vi "CD Engine lvlib.vi"(9 "Action":T1) -> (1 "Output":string)   [LabVIEW 2015, in "NIVS_Consolidated_CDW_MetaDataObj.lvclass"]
doc: "Constants, which are necessary for the <B>CD Engine library</B> in the generated custom device project."
uses:
  NIVS_Consolidated_CDW_MetaDataObj.lvclass
  CD Engine lvlib.ctl
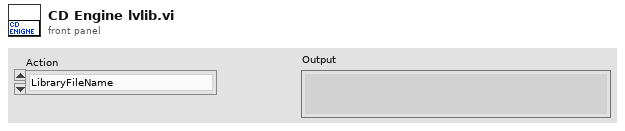
[diagram p1: front panel]
types:
  T1 = typedef "NIVS_Consolidated_CDW_MetaDataObj.lvclass/CD Engine lvlib.ctl" = enum16{"LibraryFileName", "LibraryFolderName", "Engine.FolderName", "Engine.Init.FolderName", "Engine.Run.FolderName", "Engine.Shutdown.FolderName", "Types.FolderName", "Engine.RT Driver VI.TemplatePath", "Engine.RT Driver VI.FileName", "Engine.RTStateVariables.Name", "Engine.RTStateVariables.Name.NoExtension", "Engine.Async.NameExtension", "Engine.Async.TemplateName"}
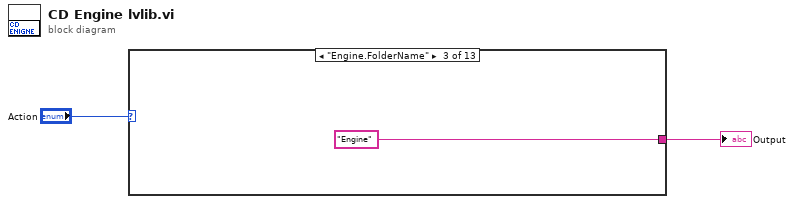
[diagram p0: block diagram]
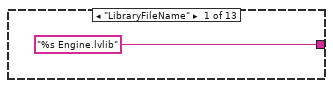
[diagram p2: hidden frame]
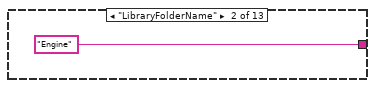
[diagram p3: hidden frame]
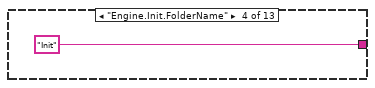
[diagram p4: hidden frame]
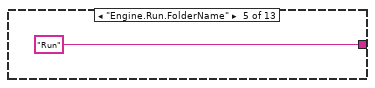
[diagram p5: hidden frame]
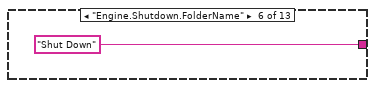
[diagram p6: hidden frame]
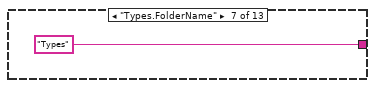
[diagram p7: hidden frame]
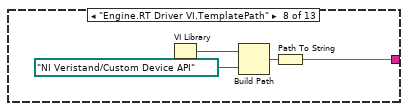
[diagram p8: hidden frame]
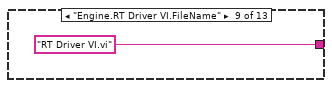
[diagram p9: hidden frame]
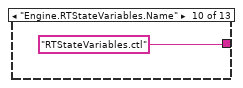
[diagram p10: hidden frame]
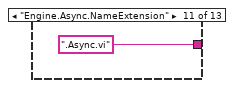
[diagram p11: hidden frame]
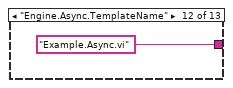
[diagram p12: hidden frame]
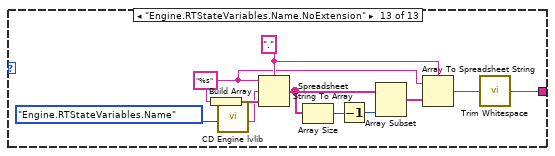
[diagram p13: hidden frame]
diagram:
  n1 = case shown="\"Engine.FolderName\"" "Action" {
    tunnel: ["%s Engine.lvlib" "Engine" "Engine" "Init" "Run" "Shut Down" "Types" w10 "RT Driver VI.vi" "RTStateVariables.ctl" ("Output") ".Async.vi" ("name or relative path") "Example.Async.vi" ("name or relative path") w18] -> w1
    frame "LibraryFileName" {
    }
    frame "LibraryFolderName" {
    }
    frame "Engine.FolderName" {
    }
    frame "Engine.Init.FolderName" {
    }
    frame "Engine.Run.FolderName" {
    }
    frame "Engine.Shutdown.FolderName" {
    }
    frame "Types.FolderName" {
    }
    frame "Engine.RT Driver VI.TemplatePath" {
      n2 = VI Library() -> (path=w11:path)
      n3 = Build Path(base path=w11, name or relative path=path "NI Veristand/Custom Device API") -> (appended path=w13:path)
      n4 = Path To String(path=w13) -> (string=w10:string)
    }
    frame "Engine.RT Driver VI.FileName" {
    }
    frame "Engine.RTStateVariables.Name" {
    }
    frame "Engine.Async.NameExtension" {
    }
    frame "Engine.Async.TemplateName" {
    }
    frame "Engine.RTStateVariables.Name.NoExtension" {
      w23 = "." ("delimiter (Tab)")
      w22 = "%s" ("format string")
      n5 = Build Array(w22) -> (w28:string[])
      n6 = call "CD Engine lvlib.vi"("Action"=CD_Engine_lvlib."Engine.RTStateVariables.Name") -> ("Output"=w20:string)  [unwired: 10 in]
      n7 = Spreadsheet String To Array(delimiter (Tab)=w23, format string=w22, spreadsheet string=w20, array type (2D Dbl)=w28) -> (array=w27:string[])
      n8 = Array Size(array=w27) -> (size(s)=w26:i32)
      n9 = Decrement(x=w26) -> (x-1=w25:i32)
      n10 = Array Subset(array=w27, length=w25) -> (w24:string[])  [unwired: 1 in]
      n11 = Array To Spreadsheet String(delimiter (Tab)=w23, array=w24, 3:w22) -> (spreadsheet string=w19:string)
      n12 = call <vilib>:"Trim Whitespace.vi"("string"=w19) -> ("trimmed string"=w18:string)  [unwired: 1 in]
    }
  }
  "Output" <- w1
